vi "ILC_servo.vi"() -> ()   [LabVIEW 2018]
uses:
  <vilib>/Simulation/Scripting/Companion Diagram/SimConfigNode/SimParams.ctl
  <vilib>/Simulation/Scripting/Companion Diagram/SimConfigNode/_simSolvers.ctl
  <vilib>/Simulation/Implementation/Shared/SIMSCR Execution Mode.ctl
  <vilib>/Simulation/Param Hierarchy/Typedefs/SIMPH Param Control Actions.ctl
  <vilib>/imath/engines/lvmath/Plug In/_Char/NIMS_CH_character datatype.ctl
  <vilib>/Simulation/Implementation/Shared/NILVSim_ParamChanged.vi
  <vilib>/Simulation/Implementation/Shared/NILVSIM_BeginStep.vi
  <vilib>/Simulation/SignalDisplay/Implementation/NILVSim Time Waveform.llb/SIM Time Waveform (vector).vi
  <vilib>/Simulation/Implementation/Shared/NILVSim_Manager.vi
  <vilib>/Utility/error.llb/Clear Errors.vi
  <vilib>/Simulation/Implementation/Shared/NILVSim_FinalizeModel.vi
  <vilib>/Simulation/Implementation/Shared/SIM Unbundle Sim Info.vi
  <vilib>/Simulation/Implementation/Shared/NILVSim_Initialize.vi
  <vilib>/addons/Control Design/_Model Construction/Model Creation.llb/CD Construct State-Space Model.vi
  <vilib>/addons/Control Design/_Model Construction/Model Creation.llb/Model Creation SubVI/cd_Create State Space Model.vi
  <vilib>/addons/Control Design/_Model Construction/Model Information.llb/CD Set Names to Model.vi
  <vilib>/addons/Control Design/_Model Construction/Model Information.llb/Model Information SubVIs/cd_Set Names To SS Model.vi
  <vilib>/addons/Control Design/_Utility/Model Viewer.llb/CD Draw State-Space Equation.vi
  <vilib>/addons/Control Design/_Utility/Model Viewer.llb/Model Viewer SubVI/cd_Draw State-Space Equation (SS).vi
  <vilib>/addons/Control Design/_Model Conversions/Continuous and Discrete.llb/CD Convert Continuous to Discrete.vi
  <vilib>/addons/Control Design/_Model Conversions/Continuous and Discrete.llb/Continuous and Discrete SubVI/cd_Convert Continuous to Discrete (SS).vi
  <vilib>/imath/engines/lvmath2/RunTimeEngine/RangeToken/NIMS_Range_R2 - Integer.vi
  <instcachedir>/0/NIMS_Range_R2 - Integer_E35B921DECF84AADB7325A02D418BFCC.lvgen/NIMS_Range_R2 - Integer_E35B921DECF84AADB7325A02D418BFCC_000.vi
  <vilib>/imath/engines/lvmath2/RunTimeEngine/CommandStatement/MC_CommandStatement_break.vi
  <vilib>/imath/engines/lvmath2/RunTimeEngine/ArithmeticOperatorToken/NIMS_ArithmeticOperator_powermx(M,M).vi
  <vilib>/imath/engines/lvmath2/RunTimeEngine/ArithmeticOperatorToken/NIMS_ArithmeticOperator_multmx.vi
  <instcachedir>/0/NIMS_ArithmeticOperator_multmx_622CA76F9646436AB036D42A9A1CE0E6.lvgen/NIMS_ArithmeticOperator_multmx_622CA76F9646436AB036D42A9A1CE0E6_006.vi
  <instcachedir>/0/NIMS_ArithmeticOperator_multmx_622CA76F9646436AB036D42A9A1CE0E6.lvgen/NIMS_ArithmeticOperator_multmx_622CA76F9646436AB036D42A9A1CE0E6_007.vi
  <vilib>/imath/engines/lvmath2/RunTimeEngine/IndexReplace/NIMS M(S,S)=M.vi
  <instcachedir>/0/NIMS M(S,S)=M_108123BD102042CF82FCAC270CFA797C.lvgen/NIMS M(S,S)=M_108123BD102042CF82FCAC270CFA797C_000.vi
  <vilib>/imathl/engines/lvmath/Functions/Error Handling/Create Error.vi
  <vilib>/imath/engines/lvmath2/RunTimeEngine/ErrorHandling/NIMS_Create Error From Enums.vi
  <vilib>/imath/engines/lvmath2/RunTimeEngine/RangeToken/NIMS_Range.vi
  <instcachedir>/0/NIMS_Range_846134F467D14A349F7C6CCEF459CDB2.lvgen/NIMS_Range_846134F467D14A349F7C6CCEF459CDB2_000.vi
  <vilib>/imath/engines/lvmath2/RunTimeEngine/BuiltInFunctions/size/NIMS_I32Row=size(GM).vi
  <instcachedir>/0/NIMS_I32Row=size(GM)_10ACDCB9F1F84A7E9F42C91D87611FB5.lvgen/NIMS_I32Row=size(GM)_10ACDCB9F1F84A7E9F42C91D87611FB5_005.vi
  <vilib>/imath/engines/lvmath2/RunTimeEngine/BuiltInFunctions/eye/NIMS_M=eye(I32V).vi
  <vilib>/imath/engines/lvmath2/RunTimeEngine/NodeEndStatement/NIMS_NodeEndStatement_Output.vi
  <instcachedir>/0/NIMS_NodeEndStatement_Output_53EC0D466D134D7ABD903AC30B43404B.lvgen/NIMS_NodeEndStatement_Output_53EC0D466D134D7ABD903AC30B43404B_005.vi
  <instcachedir>/0/NIMS_NodeEndStatement_Output_53EC0D466D134D7ABD903AC30B43404B.lvgen/NIMS_NodeEndStatement_Output_53EC0D466D134D7ABD903AC30B43404B_002.vi
  <instcachedir>/0/NIMS_NodeEndStatement_Output_53EC0D466D134D7ABD903AC30B43404B.lvgen/NIMS_NodeEndStatement_Output_53EC0D466D134D7ABD903AC30B43404B_012.vi
  <instcachedir>/0/NIMS_NodeEndStatement_Output_53EC0D466D134D7ABD903AC30B43404B.lvgen/NIMS_NodeEndStatement_Output_53EC0D466D134D7ABD903AC30B43404B_003.vi
  <vilib>/imath/engines/lvmath2/RunTimeEngine/ErrorHandling/NIMS_Finalize Error.vi
  <vilib>/imath/engines/lvmath2/RunTimeEngine/BuiltInFunctions/norm/NIMS_norm(GM,DBL).vi
  <instcachedir>/0/NIMS_norm(GM,DBL)_14A9435485184B5E92336AF75A728284.lvgen/NIMS_norm(GM,DBL)_14A9435485184B5E92336AF75A728284_001.vi
  <vilib>/imath/engines/lvmath2/RunTimeEngine/IndexReplace/NIMS V(S)=S.vi
  <instcachedir>/0/NIMS V(S)=S_420DA4522869420292A92FA3CC108C4E.lvgen/NIMS V(S)=S_420DA4522869420292A92FA3CC108C4E_000.vi
  <instcachedir>/0/NIMS_ArithmeticOperator_multmx_622CA76F9646436AB036D42A9A1CE0E6.lvgen/NIMS_ArithmeticOperator_multmx_622CA76F9646436AB036D42A9A1CE0E6_011.vi
  <instcachedir>/0/NIMS_ArithmeticOperator_multmx_622CA76F9646436AB036D42A9A1CE0E6.lvgen/NIMS_ArithmeticOperator_multmx_622CA76F9646436AB036D42A9A1CE0E6_003.vi
  <vilib>/imath/engines/lvmath2/RunTimeEngine/ArithmeticOperatorToken/NIMS_ArithmeticOperator_plus.vi
  <instcachedir>/0/NIMS_ArithmeticOperator_plus_DE670E32103C4C10ADF2A97367172B30.lvgen/NIMS_ArithmeticOperator_plus_DE670E32103C4C10ADF2A97367172B30_010.vi
  <vilib>/imath/engines/lvmath2/RunTimeEngine/BuiltInFunctions/inv/NIMS_inv(GM).vi
  <instcachedir>/0/NIMS_inv(GM)_A6DF8FE880224208AACFE4CF9F659502.lvgen/NIMS_inv(GM)_A6DF8FE880224208AACFE4CF9F659502_001.vi
  <instcachedir>/0/NIMS_ArithmeticOperator_plus_DE670E32103C4C10ADF2A97367172B30.lvgen/NIMS_ArithmeticOperator_plus_DE670E32103C4C10ADF2A97367172B30_002.vi
  <vilib>/imath/engines/lvmath2/RunTimeEngine/ArithmeticOperatorToken/NIMS_ArithmeticOperator_minus.vi
  <instcachedir>/0/NIMS_ArithmeticOperator_minus_C4D0373119CC411691B2E50DF2E09F22.lvgen/NIMS_ArithmeticOperator_minus_C4D0373119CC411691B2E50DF2E09F22_009.vi
  <vilib>/Simulation/Utility/Implementation/NILVSim Get Time and IsAcceptedStep.vi
  <vilib>/Simulation/Implementation/Shared/SIMSH Read Queue.vi
  <vilib>/Simulation/Implementation/Shared/NILVSim_GetModelError.vi
  <vilib>/Simulation/Implementation/Shared/SIM Bundle Sim Info.vi
  <vilib>/imath/engines/lvmath2/RunTimeEngine/Managers/WorkSpace/UID Generator.vi
  <vilib>/imath/engines/lvmath2/RunTimeEngine/BuiltInFunctions/figure/NIMS_figure.vi
  <vilib>/imath/engines/lvmath2/RunTimeEngine/BuiltInFunctions/plot/NIMS_plot(RM, RM, Str).vi
  <vilib>/imath/engines/lvmath/Plug In/_Char/NIMS_CH_Character RV to String.vi
  <vilib>/imath/engines/lvmath2/RunTimeEngine/BuiltInFunctions/xlabel/NIMS_xlabel.vi
  <vilib>/imath/engines/lvmath2/RunTimeEngine/BuiltInFunctions/ylabel/NIMS_ylabel.vi
  <instcachedir>/0/NIMS_Range_846134F467D14A349F7C6CCEF459CDB2.lvgen/NIMS_Range_846134F467D14A349F7C6CCEF459CDB2_001.vi
  <vilib>/imath/engines/lvmath2/RunTimeEngine/Managers/SymbolTable/Clear UID.vi
  <vilib>/Simulation/Scripting/Companion Diagram/SimConfigNode/SimDog.xnode
  <vilib>/Simulation/Implementation/XNodeFramework/SimXNode/SimX.xnode
  <vilib>/addons/Control Design/_Model Conversions/NI_CD_Continuous and Discrete.lvlib
  <vilib>/addons/Control Design/_Model Construction/NI_LinSys_Model Creation.lvlib
  <vilib>/addons/Control Design/_Model Construction/NI_LinSys_Model Information.lvlib
  <vilib>/addons/Control Design/_Utility/NI_CD_Model Viewer.lvlib
  <vilib>/Simulation/Implementation/Shared/NI_SIM_Implementation.lvlib
  <vilib>/imath/engines/lvmath2/RunTimeEngine/Managers/SymbolTable/NIMS_WorkSpace.lvlib
panel:
  out "XY Graph 3":cdb[](graph)
  out "Waveform Chart":waveform(dbl)[](graph)
  out "XY Graph 2":cdb[](graph)
  out "Error":errorcluster
  out "Equation":picture
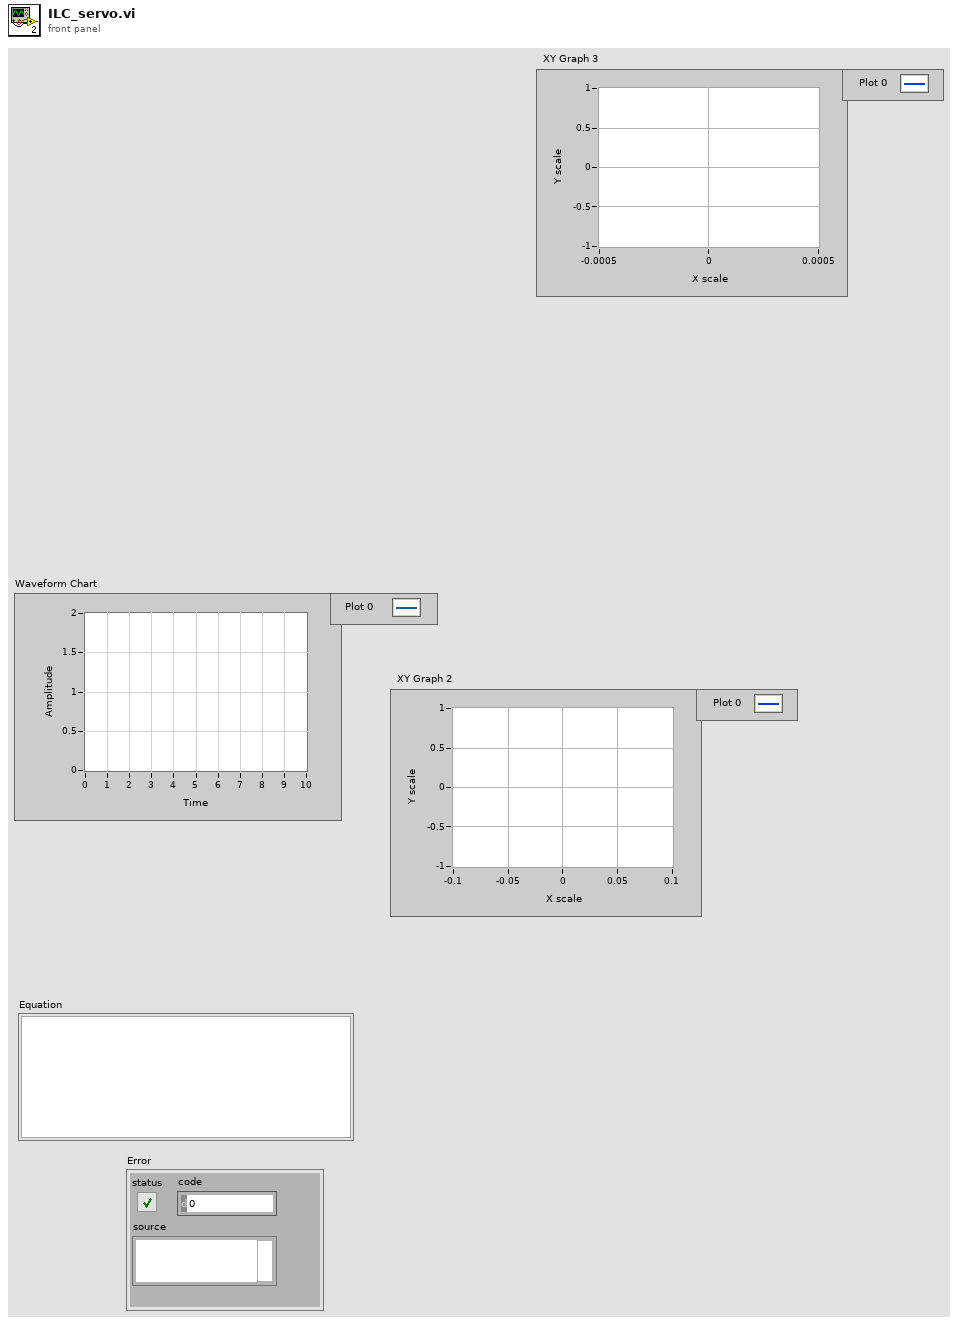
[diagram p1: front panel]
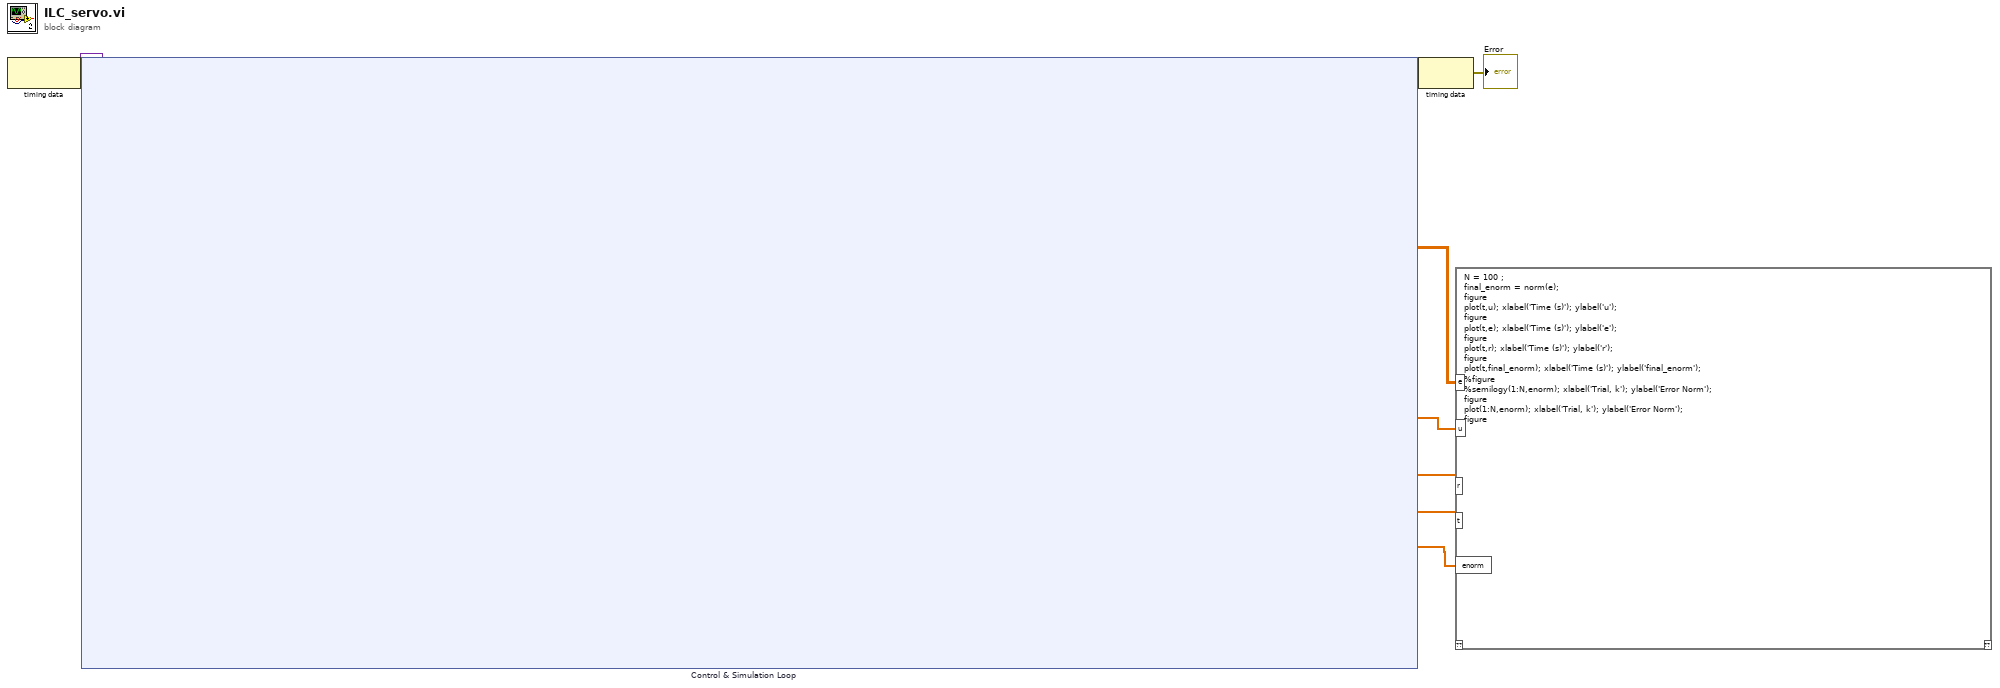
[diagram p0: block diagram]
diagram:
  n1 = node-c288() -> (w8:variant)  [unwired: 1 in]
  n2 = node-c254 "Control & Simulation Loop"(w8) -> (w7:variant, w5:dbl[], w4:dbl[], w3:cdb[][], w2:cdb[], w1:dbl[])
  n3 = node-c288(w7) -> (→"Error":errorcluster)
  n4 = mathscript code="N = 100 ;\nfinal_enorm = norm(e);\nfigure\nplot(t,u); xlabel('Time (s)'); ylabel('u');\nfigure\nplot(t,e); xlabel('Time (s)'); ylabel('e');\nfigure\nplot(t,r); xlabel('Time (s)'); ylabel('r');\nfigure\nplot(t,final_enorm); xlabel('Time (s)'); ylabel('final_enorm');\n%figure\n%semilogy(1:N,enorm); xlabel('Trial, k'); ylabel('Error Norm');\nfigure\nplot(1:N,enorm); xlabel('Trial, k'); ylabel('Error Norm');\nfigure" ("MathScript Node 2")("r"=w4, "t"=w5, "u"=w2, "e"=w3, "enorm"=w1) -> ()  [unwired: 1 in, 1 out]
